vi "load_plot_window_dyn.vi"(8 "error in (no error)":errorcluster, 11 "Plots in":refnum<class "Plots.lvclass">) -> (0 "error out":errorcluster, 3 "Plots out":refnum<class "Plots.lvclass">)   [LabVIEW 2017, in "Plots.lvclass"]
doc: "loads a new plot window dynalically"
uses:
  Plots.lvclass
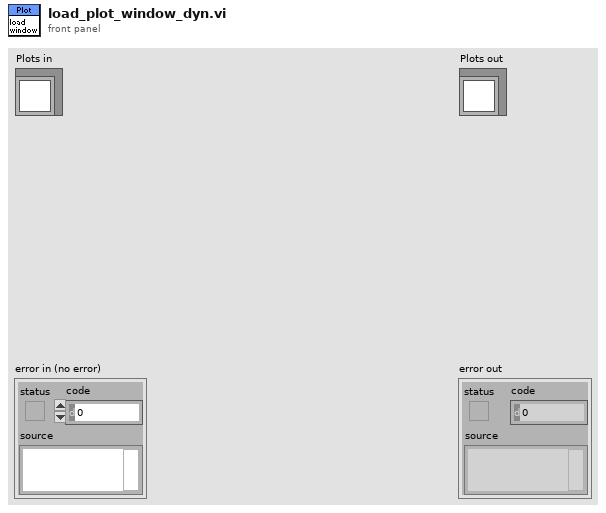
[diagram p1: front panel]
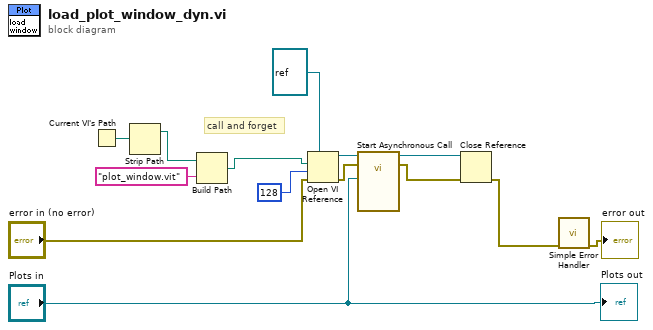
[diagram p0: block diagram]
diagram:
  # "call and forget"
  n1 = Current VI's Path() -> (path=w3:path)
  n2 = Strip Path(path=w3) -> (stripped path=w4:path)  [unwired: 1 out]
  n3 = Build Path(base path=w4, name or relative path="plot_window.vit") -> (appended path=w1:path)
  n4 = Open VI Reference(type specifier VI Refnum (for type only)=refnum<vi> refnum, vi path=w1, options=128, error in (no error)="error in (no error)") -> (vi reference=w5:refnum<vi>, error out=w8:errorcluster)  [unwired: 2 in]
  n5 = call-by-ref "Start Asynchronous Call"(reference=w5, error in=w8, "Plots in"="Plots in") -> (reference out=w10:refnum<vi>, error out=w9:errorcluster)  [unwired: 9 in, 2 out]
  n6 = Close Reference(reference=w10, error in (no error)=w9) -> (error out=w7:errorcluster)
  n7 = call <vilib>:"Simple Error Handler.vi"("error in (no error)"=w7) -> ("error out"=→"error out":errorcluster)  [unwired: 4 in, 4 out]
  "Plots out" <- "Plots in"
